vi "Waveform Attribute, Append Array.vi"(6 "error in":errorcluster, 7 "value":dbl=nan, 8 "label":string="my label", 9 "attributes":T1[](array[typedef]) {"Value" format="%#.3f"}) -> (0 "error out":errorcluster, 3 "attributes out":T1[](array[typedef]) {"Value" format="%#.3f"})   [LabVIEW 2010]
doc: "This function gets all of the waveform attribute labels and values using a control reference.\n\nAny waveform attributes that will not convert to double precision floating point numbers will be set to NaN."
uses:
  Waveform Attribute Cluster.ctl
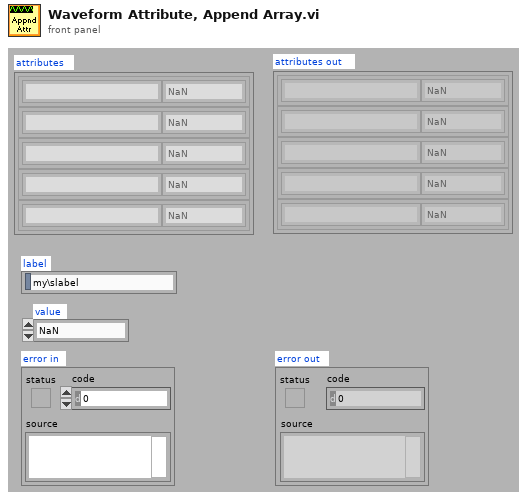
[diagram p1: front panel]
types:
  T1 = typedef "Waveform Attribute Cluster.ctl" = cluster{"Label":string, "Value":dbl}
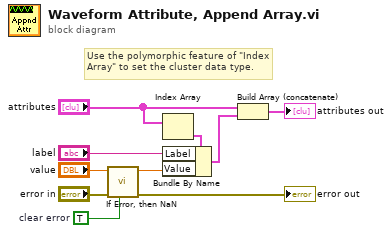
[diagram p0: block diagram]
diagram:
  w3 = TRUE  # clear error
  # "Use the polymorphic feature of \"Index Array\" to set the cluster data type."
  n1 = call "If Error, then NaN.vi"("clear error (F)"=w3, "error in (T)"="error in", "value1"="value") -> ("error out"=→"error out":errorcluster, "value out1"=w1:dbl)  [unwired: 3 in, 2 out]
  n2 = Index Array(array="attributes") -> (element=w6:T1)  [unwired: 1 in]
  n3 = Bundle By Name(cluster=w6, "Label"="label", "Value"=w1) -> (w7:T1)
  n4 = Build Array (concatenate)("attributes", w7) -> (→"attributes out":T1[])
